vi "IIC Get Slave Addr.vi"(9 "pSlaveAddr":i16[](array[numeric])=[0, 0, 0, 0, 0, 0, 0, 0, 0, 0, 0, 0, 0, 0, 0, 0, 0, 0, 0, 0, 0, 0, 0, 0, 0, 0, 0, 0, 0, 0, 0, 0, 0, 0, 0, 0, 0, 0, 0, 0, 0, 0, 0, 0, 0, 0, 0, 0, 0, 0, 0, 0, 0, 0, 0, 0, 0, 0, 0, 0, 0, 0, 0, 0, 0, 0, 0, 0, 0, 0, 0, 0, 0, 0, 0, 0, 0, 0, 0, 0, 0, 0, 0, 0, 0, 0, 0, 0, 0, 0, 0, 0, 0, 0, 0, 0, 0, 0, 0, 0, 0, 0, 0, 0, 0, 0, 0, 0, 0, 0, 0, 0, 0, 0, 0, 0, 0, 0, 0, 0, 0, 0, 0, 0, 0, 0, 0, 0], 10 "IICIndex":i32, 11 "DevHandle":i32) -> (1 "pSlaveAddr out":i16[](array[numeric]), 3 "function return":i32)   [LabVIEW 2010, in "usb2iic.lvlib"]
doc: "int WINAPI IIC_GetSlaveAddr(int DevHandle,int IICIndex,short *pSlaveAddr);"
uses:
  usb2iic.lvlib
  USB2XXX.dll
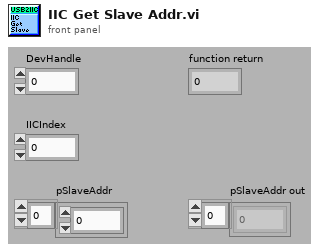
[diagram p1: front panel]
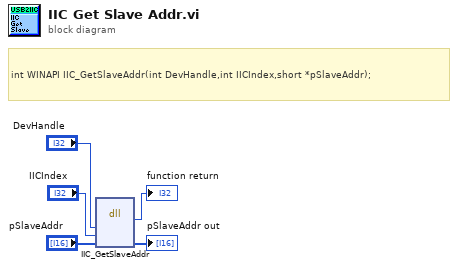
[diagram p0: block diagram]
diagram:
  # "int WINAPI IIC_GetSlaveAddr(int DevHandle,int IICIndex,short *pSlaveAddr);"
  n1 = dll-call lib="G:/OtherWork/USB2XXX_Example/trunk/Labview/PublicFiles/USB2XXX.*" fn="IIC_GetSlaveAddr"("DevHandle"="DevHandle", "IICIndex"="IICIndex", "pSlaveAddr"="pSlaveAddr") -> (→"function return":i32, "pSlaveAddr"=→"pSlaveAddr out":i16[])  [unwired: 5 in, 2 out]
